vi "Get SplitterRef.vi"(8 "error in":errorcluster caption="错误输入（无错误）", 11 "PanelDataNode 输入":refnum<class "PanelDataNode.lvclass"> caption="DNL_LabVIEW Object in") -> (0 "error out":errorcluster caption="错误输出", 2 "Splitter":refnum<vi>, 3 "PanelDataNode 输出":refnum<class "PanelDataNode.lvclass"> caption="DNL_LabVIEW Object out")   [LabVIEW 2016, in "PanelDataNode.lvclass"]
uses:
  PanelDataNode.lvclass
  PanelDataNode.lvclass/PanelDataNode.ctl
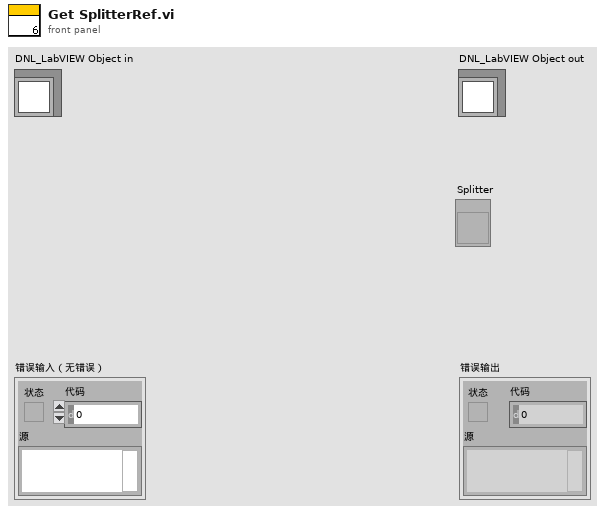
[diagram p1: front panel]
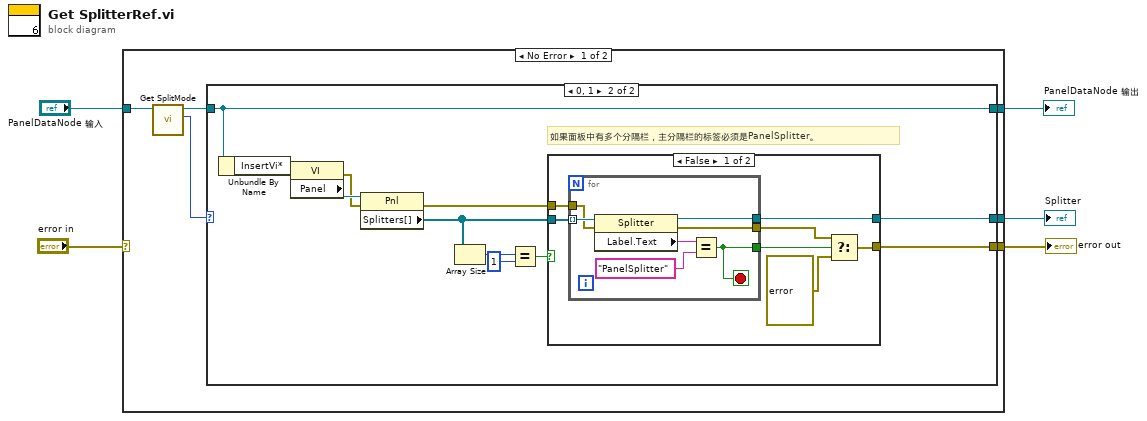
[diagram p0: block diagram]
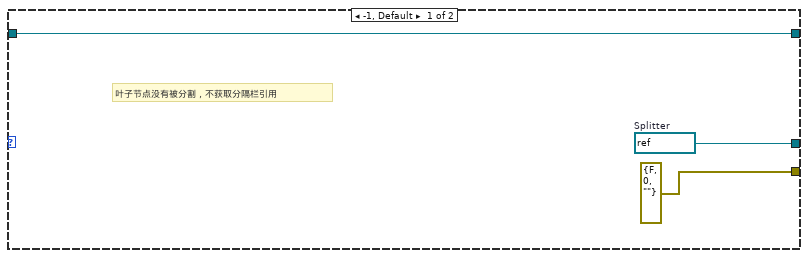
[diagram p2: hidden frame]
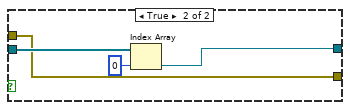
[diagram p3: hidden frame]
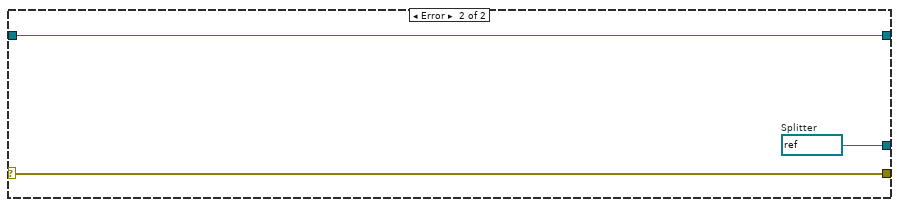
[diagram p4: hidden frame]
diagram:
  n1 = case shown="No Error" "error in" {
    selector: "error in" -> [_ w46]
    tunnel: [w6 w45] -> w3
    tunnel: "PanelDataNode 输入" -> [w11 w45]
    tunnel: [w8 w46] -> w2
    tunnel: [w7 w44] -> w1
    frame No Error {
      n2 = call-dynamic "Get SplitMode.vi"("PanelDataNode 输入"=w11) -> ("Split Mode"=w9:i32, "PanelDataNode 输出"=w10:refnum<class "PanelDataNode.lvclass">)  [unwired: 8 in, 1 out]
      n3 = case shown="0, 1" w9 {
        tunnel: w10 -> [w12 w15]
        tunnel: [w13 w17] -> w7
        tunnel: [errorcluster {"status"=FALSE, "code"=0, "source"=""} ("error out") w16] -> w8
        tunnel: [w12 w15] -> w6
        frame -1, Default {
          w13 = refnum<vi> refnum  # Splitter
          # "叶子节点没有被分割，不获取分隔栏引用"
        }
        frame 0, 1 {
          # "如果面板中有多个分隔栏，主分隔栏的标签必须是PanelSplitter。"
          n4 = Unbundle By Name(w15) -> ("InsertVi*"=w24:refnum<vi>)
          n5 = property class="VI"(reference=w24) -> (error out=w19:errorcluster, "Panel"=w25:refnum<vi>)  [unwired: 1 in, 1 out]
          n6 = property class="Pnl"(reference=w25, error in=w19) -> (error out=w18:errorcluster, "Splitters[]"=w20:refnum<vi>[])  [unwired: 1 out]
          n7 = Array Size(array=w20) -> (size(s)=w23:i32)
          n8 = Equal?(x=w23, y=1) -> (x = y?=w21:bool)
          n9 = case shown="False" w21 {
            tunnel: w20 -> [w32 w43]
            tunnel: [w30 w41] -> w17
            tunnel: w18 -> [w31 w40]
            tunnel: [w26 w40] -> w16
            frame False {
              n10 = for {
                tunnel: w32 -> [w39] mode=indexing
                tunnel: [w36] -> w30
                tunnel: w31 -> [w35]
                tunnel: [w34] -> w28
                tunnel: [w33] -> w29
                stop <- w33 stop-if-true
                n11 = property class="Splitter"(reference=w39, error in=w35) -> (reference out=w36:refnum<vi>, error out=w34:errorcluster, "Label.Text"=w38:string)
                n12 = Equal?(x=w38, y="PanelSplitter") -> (x = y?=w33:bool)
              }
              n13 = Select(t=w28, s=w29, f=errorcluster {"status"=TRUE, "code"=0, "source"="无法找到分隔栏！如果面板中有多个分隔栏，请将主分隔栏标签设置为PanelSplitter。"}) -> (s? t:f=w26:errorcluster)
            }
            frame True {
              n14 = Index Array(array=w43, index=0 ("索引")) -> (element=w41:refnum<vi>)
            }
          }
        }
      }
    }
    frame Error {
      w44 = refnum<vi> refnum  # Splitter
    }
  }
  "error out" <- w2
  "PanelDataNode 输出" <- w3
  "Splitter" <- w1
